vi "Delete_First_Rows.vi"(2 "Data In":string[][](array[string]), 3 "File Type":string) -> (0 "Data Out":string[][](array[string]), 1 "Rows removed":i32)   [LabVIEW 2010]
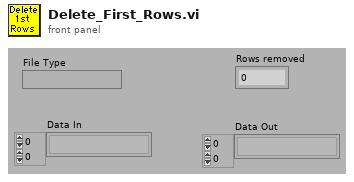
[diagram p1: front panel]
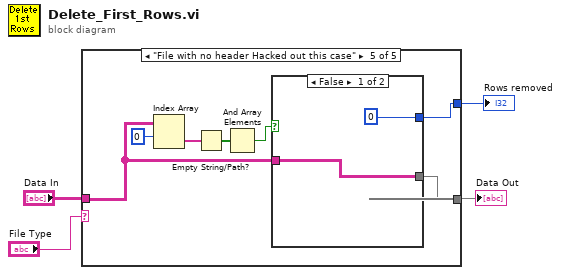
[diagram p0: block diagram]
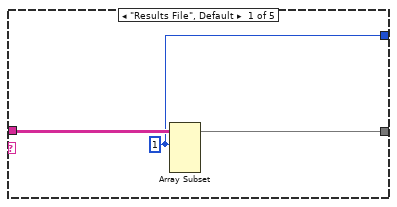
[diagram p2: hidden frame]
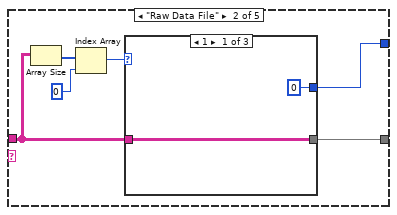
[diagram p3: hidden frame]
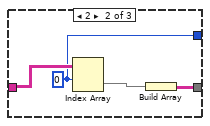
[diagram p4: hidden frame]
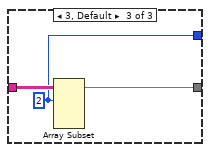
[diagram p5: hidden frame]
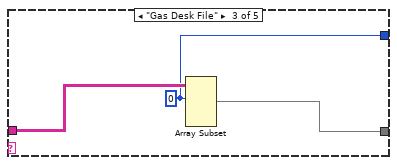
[diagram p6: hidden frame]
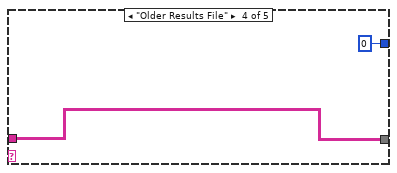
[diagram p7: hidden frame]
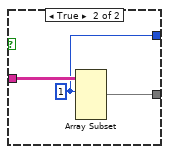
[diagram p8: hidden frame]
diagram:
  n1 = case shown="\"File with no header Hacked out this case\"" "File Type" {
    tunnel: [w6 w13 w24 w27 w30] -> w4
    tunnel: "Data In" -> [w7 w11 w25 w27 w31]
    tunnel: [w5 w8 w23 0 ("Array Index") w28] -> w1
    frame "Results File", Default {
      w5 = 1 ("Array Index")
      n2 = Array Subset(array=w7, index (row)=w5) -> (w6:string[][])  [unwired: 3 in]
    }
    frame "Raw Data File" {
      n3 = Array Size(array=w11) -> (size(s)=w12:i32[])
      n4 = Index Array(array=w12, index=0 ("Index")) -> (element=w9:i32)
      n5 = case shown="1" w9 {
        tunnel: [w15 w17 w22] -> w13
        tunnel: w11 -> [w15 w19 w21]
        tunnel: [0 w16 w20] -> w8
        frame 1 {
        }
        frame 2 {
          w16 = 0 ("Index")
          n6 = Index Array(array=w19, index (row)=w16) -> (element=w18:string[])  [unwired: 1 in]
          n7 = Build Array(w18) -> (w17:string[][])
        }
        frame 3, Default {
          w20 = 2 ("Array Index")
          n8 = Array Subset(array=w21, index (row)=w20) -> (w22:string[][])  [unwired: 3 in]
        }
      }
    }
    frame "Gas Desk File" {
      w23 = 0 ("Array Index")
      n9 = Array Subset(array=w25, index (row)=w23) -> (w24:string[][])  [unwired: 3 in]
    }
    frame "Older Results File" {
    }
    frame "File with no header Hacked out this case" {
      n10 = Index Array(array=w31, index (row)=0) -> (element=w33:string[])  [unwired: 1 in]
      n11 = Empty String/Path?(string/path=w33) -> (empty?=w32:bool[])
      n12 = And Array Elements(Boolean array=w32) -> (logical AND=w29:bool)
      n13 = case shown="False" w29 {
        tunnel: w31 -> [w35 w39]
        tunnel: [w35 w38] -> w30
        tunnel: [0 ("Array Index") w37] -> w28
        frame False {
        }
        frame True {
          w37 = 1 ("Array Index")
          n14 = Array Subset(array=w39, index (row)=w37) -> (w38:string[][])  [unwired: 3 in]
        }
      }
    }
  }
  "Data Out" <- w4
  "Rows removed" <- w1
